vi "Put Serial Str V.vi"(8 "error in (no error)":errorcluster, 11 "stringtoport":string) -> (0 "error out":errorcluster, 2 "function return":i16, 3 "stringtoport out":string)   [LabVIEW 2009, in "VantagePro.lvlib"]
doc: "DllAccess short int _stdcall PutSerialStr_V (char *stringtoport);"
uses:
  VantagePro.lvlib
  <userlib>/VantagePro/VantagePro.dll
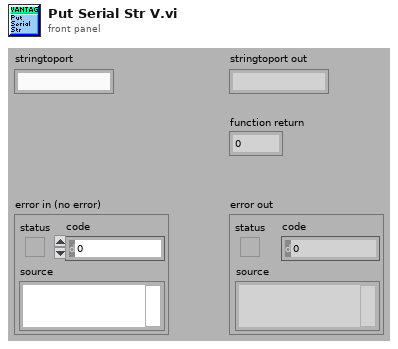
[diagram p1: front panel]
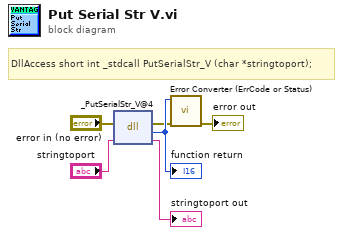
[diagram p0: block diagram]
diagram:
  # "DllAccess short int _stdcall PutSerialStr_V (char *stringtoport);"
  n1 = dll-call lib="C:/Program Files/National Instruments/LabVIEW 2010/user.lib/VantagePro/VantagePro.*" fn="_PutSerialStr_V@4"(error in="error in (no error)", "stringtoport"="stringtoport") -> (error out=w2:errorcluster, w6:i16, "stringtoport"=→"stringtoport out":string)  [unwired: 2 in, 1 out]
  "function return" <- w6
  n2 = call "Error Converter (ErrCode or Status).vi"("error in (no error)"=w2, "error code"=w6) -> ("error out"=→"error out":errorcluster)  [unwired: 9 in]
